vi "FGV - Attocube Actions.vi"(4 "error in":errorcluster, 6 "Function":enum16{"write", "read"}(ring), 7 "Actions IN":T1) -> (0 "error out":errorcluster, 3 "Actions OUT":T1)   [LabVIEW 2013]
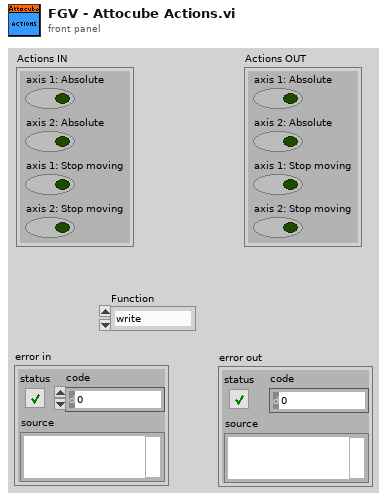
[diagram p1: front panel]
types:
  T1 = cluster{"axis 1: Absolute":bool, "axis 2: Absolute":bool, "axis 1: Stop moving":bool, "axis 2: Stop moving":bool}
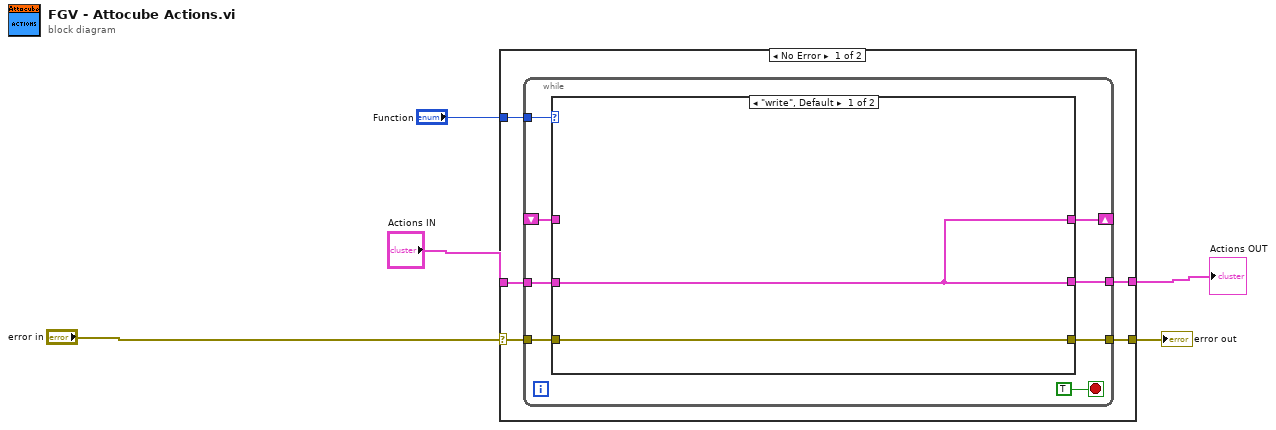
[diagram p0: block diagram]
diagram:
  n1 = case shown="No Error" "error in" {
    selector: "error in" -> [w10 w24]
    tunnel: [w9 w24] -> w5
    tunnel: [w8 w23] -> w3
    tunnel: "Function" -> [w7 _]
    tunnel: "Actions IN" -> [w6 w23]
    frame No Error {
      n2 = while {
        shift-right: [w13] -> _
        shift-left: _ -> [w12]
        tunnel: w10 -> [w17]
        tunnel: [w16] -> w9
        tunnel: [w15] -> w8
        tunnel: w7 -> [w14]
        tunnel: w6 -> [w11]
        stop <- TRUE stop-if-true
        n3 = case shown="\"write\", Default" w14 {
          tunnel: w17 -> [w19 w21]
          tunnel: [w19 w21] -> w16
          tunnel: [w20 w22] -> w15
          tunnel: [w20 w22] -> w13
          tunnel: w12 -> [_ w22]
          tunnel: w11 -> [w20 _]
          frame "write", Default {
          }
          frame "read" {
          }
        }
      }
    }
    frame Error {
    }
  }
  "error out" <- w5
  "Actions OUT" <- w3
